vi "UDP_Clientei.vi"() -> ()   [LabVIEW 2020]
panel:
  in  "stop 2":bool
  in  "Puerto de Destino":u16
  in  "String":string
  out "data out":string
  in  "stop":bool
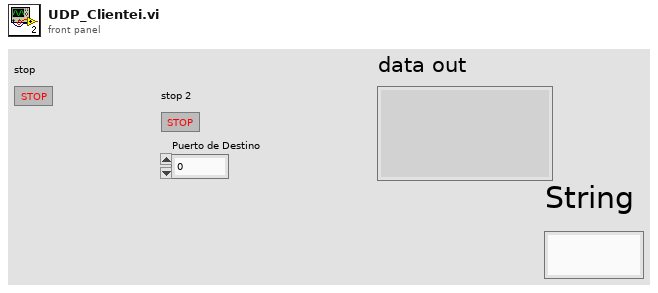
[diagram p1: front panel]
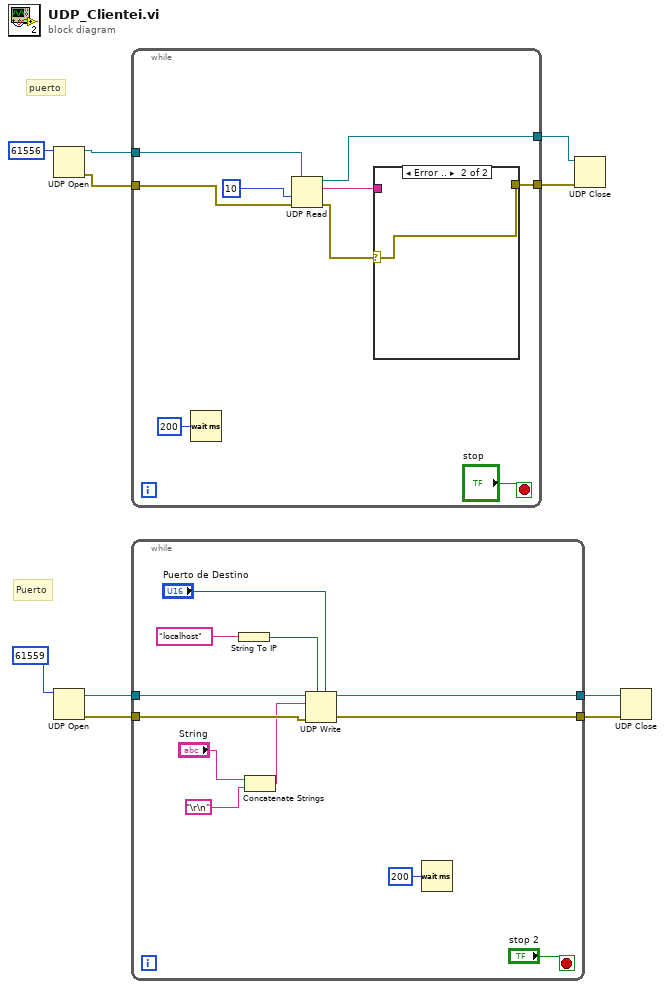
[diagram p0: block diagram]
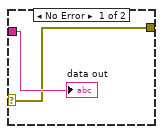
[diagram p2: hidden frame]
diagram:
  # "Puerto"
  # "puerto"
  n1 = UDP Open(11:u16 61556 ("port")) -> (port=w9:refnum<k16>, 0:w8:errorcluster)  [unwired: 4 in, 1 out]
  n2 = UDP Open(11:u16 61559 ("port")) -> (port=w4:refnum<k16>, 0:w3:errorcluster)  [unwired: 4 in, 1 out]
  n3 = while {
    tunnel: w9 -> [w18]
    tunnel: w8 -> [w17]
    tunnel: [w14] -> w7
    tunnel: [w12] -> w6
    stop <- "stop" stop-if-true
    n4 = Wait (ms)(milliseconds to wait=u32 200) -> ()  [unwired: 1 out]
    n5 = UDP Read(connection ID=w18, timeout ms (25000)=10, 8:w17) -> (data out=w13:string, error out=w15:errorcluster, 3:w14:refnum<k16>)  [unwired: 1 in, 2 out]
    n6 = case shown="Error .." w15 {
      selector: w15 -> [w20 w22]
      tunnel: w13 -> [w21 _]
      tunnel: [w20 w22] -> w12
      frame No Error {
        "data out" <- w21
      }
      frame Error {
      }
    }
  }
  n7 = while {
    tunnel: w4 -> [w33]
    tunnel: w3 -> [w32]
    tunnel: [w26] -> w2
    tunnel: [w25] -> w1
    stop <- "stop 2" stop-if-true
    n8 = String To IP(1:"localhost") -> (0:w31:u32)
    n9 = Concatenate Strings("String", "\r\n") -> (w28:string)
    n10 = UDP Write(address=w31, port or service name="Puerto de Destino", connection ID=w33, data in=w28, 8:w32) -> (error out=w25:errorcluster, 3:w26:refnum<k16>)  [unwired: 1 in]
    n11 = Wait (ms)(milliseconds to wait=u32 200) -> ()  [unwired: 1 out]
  }
  n12 = UDP Close(connection ID=w7, 8:w6) -> ()  [unwired: 2 out]
  n13 = UDP Close(connection ID=w2, 8:w1) -> ()  [unwired: 2 out]
